vi "artificial data.vi"(11 "data input":dbl[](array[numeric])) -> (3 "data input with fake date if needed":dbl[](array[numeric]))   [LabVIEW 2019]
uses:
  data channels.ctl
  <vilib>/numeric/Random Number (Range) DBL.vi
panel:
  in  "artificial data":dbl[](array[numeric])=[0.5, 0.1, 0.05, 0.0, 10.0, 1.0, 0.8, 0.3]
  out "Strings []":string[](array[string])=["plant flow [L/s]", "Head Loss [m]", "sludge flow [L/s]", "UV 254", "raw [NTU]", "floc sed [NTU]", "clarified [NTU]", "filtered [NTU]"]
  in  "channel":T1
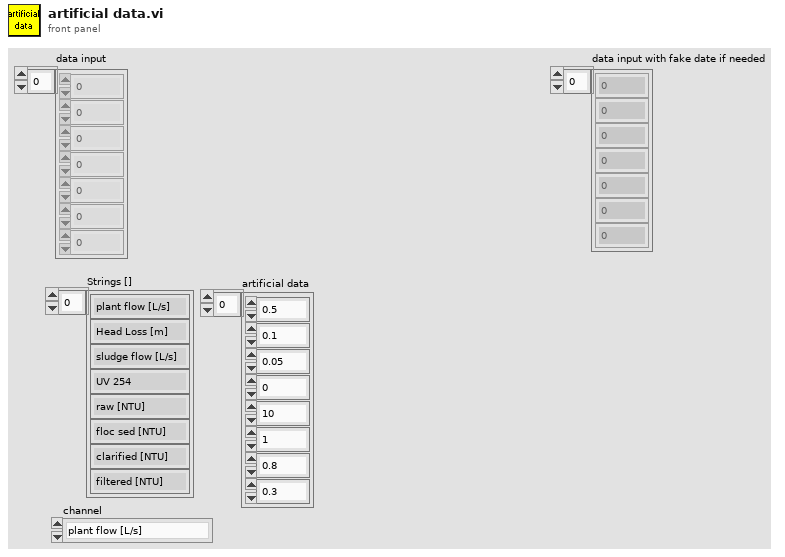
[diagram p1: front panel]
types:
  T1 = typedef "data channels.ctl" = enum16{"plant flow [L/s]", "Head Loss [m]", "sludge flow [L/s]", "UV 254", "raw [NTU]", "floc sed [NTU]", "clarified [NTU]", "filtered [NTU]"}
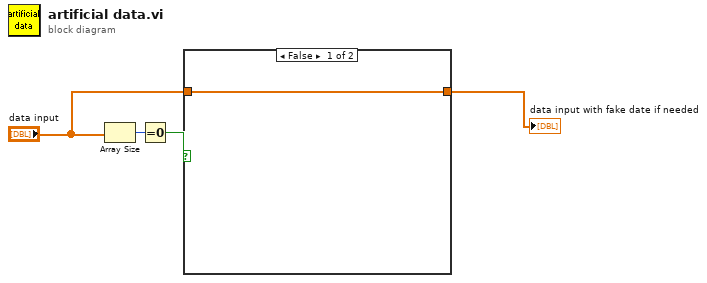
[diagram p0: block diagram]
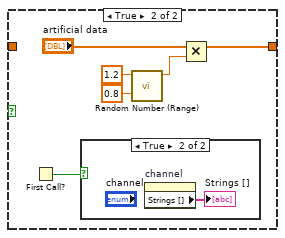
[diagram p2: hidden frame]
diagram:
  n1 = Array Size(array="data input") -> (size(s)=w4:i32)
  n2 = Equal To 0?(x=w4) -> (x = 0?=w3:bool)
  n3 = case shown="False" w3 {
    tunnel: [w5 w7] -> w2
    tunnel: "data input" -> [w5 _]
    frame False {
    }
    frame True {
      n4 = First Call?() -> (First Call?: T/F=w10:bool)
      n5 = case shown="True" w10 {
        frame False {
        }
        frame True {
          n6 = property on="channel" class="Enum (strict)"() -> ("Strings []"=→"Strings []":string[])  [unwired: 2 in, 2 out]
        }
      }
      n7 = call-poly <vilib>:"Random Number (Range).vi"("lower bound (0)"=0.8, "upper bound (100)"=1.2) -> ("number"=w6:dbl)  [unwired: 9 in]
      n8 = Multiply(x="artificial data", y=w6) -> (x*y=w7:dbl[])
    }
  }
  "data input with fake date if needed" <- w2
